vi "Init.vi"(0 "ClassReaderGOOP300 in":refnum<class "ClassReaderGOOP300.lvclass">, 1 "LvClassRef":refnum<vi>, 5 "error in (no error)":errorcluster) -> (14 "ClassReaderGOOP300 out":refnum<class "ClassReaderGOOP300.lvclass">, 19 "error out":errorcluster)   [LabVIEW 2016, in "ClassReaderGOOP300.lvclass"]
uses:
  <resource>/Framework/Providers/Open_GDS/ClassProviders/Provider_EndevoGOOP300/ClassReaderGOOP300_class/ClassReaderGOOP300.lvclass
  <resource>/Framework/Providers/Open_GDS/ClassProviders/Provider_LvNativeClass/ClassReaderNative_class/ClassReaderNative.lvclass
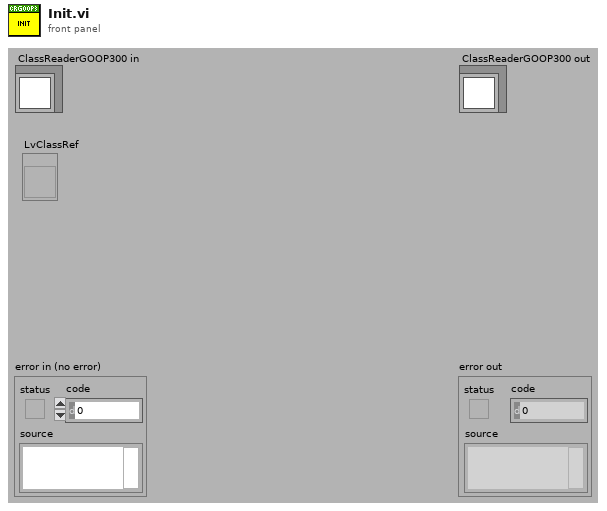
[diagram p1: front panel]
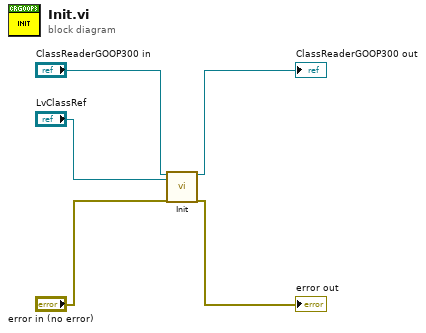
[diagram p0: block diagram]
diagram:
  n1 = call-parent "Init.vi"("ClassReaderNative in"="ClassReaderGOOP300 in", "LvClassRef"="LvClassRef", "error in (no error)"="error in (no error)") -> ("ClassReaderNative out"=→"ClassReaderGOOP300 out":refnum<class "ClassReaderGOOP300.lvclass">, "error out"=→"error out":errorcluster)  [unwired: 15 in]
